vi "New_To_Old.vi"(8 "error in":errorcluster caption="错误输入") -> (0 "error out":errorcluster caption="错误输出")   [LabVIEW 2014]
uses:
  Global_var/Global_var.vi
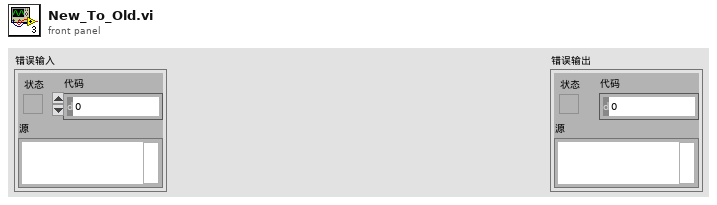
[diagram p1: front panel]
types:
  T1 = typedef "Global_Goal.ctl" = string
  T2 = typedef "Point.ctl" = cluster{"x":dbl, "y":dbl, "z":dbl}
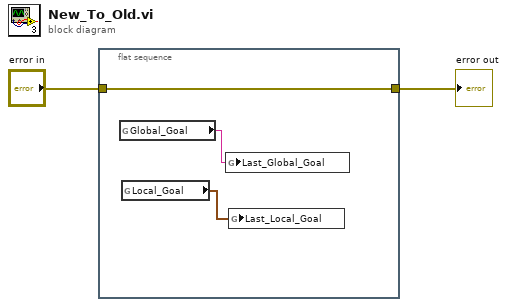
[diagram p0: block diagram]
diagram:
  n1 = flat-sequence {
    tunnel: [w3] -> w2
    tunnel: "error in" -> [w3]
    frame #0 {
      n2 = global read "Global_var.vi" "Global_Goal"() -> (w5:T1)
      n3 = global read "Global_var.vi" "Local_Goal"() -> (w4:T2)
      n4 = global write "Global_var.vi" "Last_Global_Goal"(w5) -> ()
      n5 = global write "Global_var.vi" "Last_Local_Goal"(w4) -> ()
    }
  }
  "error out" <- w2
